vi "Prompt User for Init Type.vi"(8 "error in (no error)":errorcluster) -> (0 "error out":errorcluster, 3 "Path out":path)   [LabVIEW 2019, in "FPGA Addon System Explorer.lvlib"]
uses:
  FPGA Addon System Explorer.lvlib
panel:
  in  "New Instance?":bool
  in  "OK":bool
  in  "Path":path
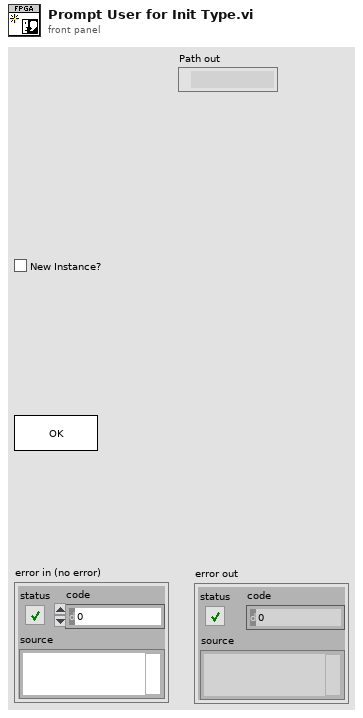
[diagram p1: front panel]
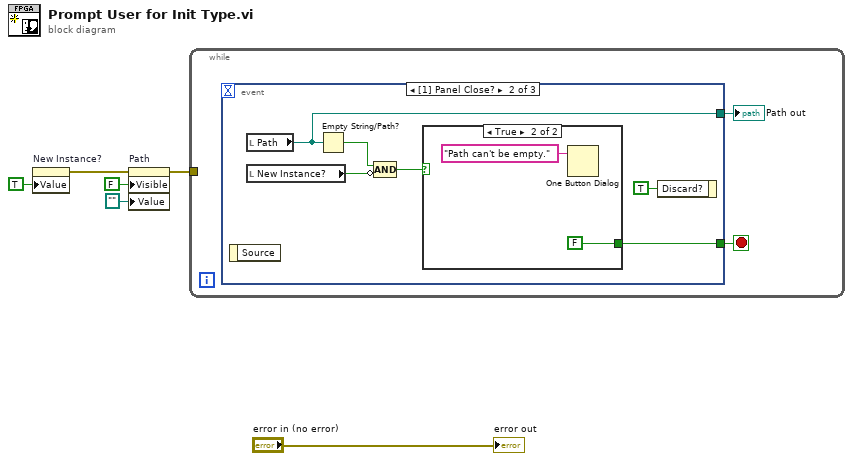
[diagram p0: block diagram]
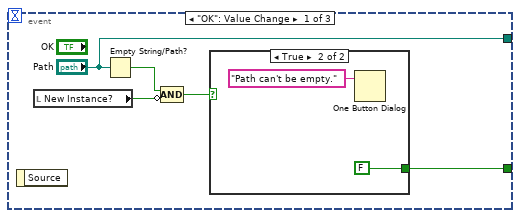
[diagram p2: hidden frame]
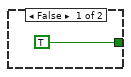
[diagram p3: hidden frame]
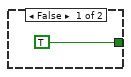
[diagram p4: hidden frame]
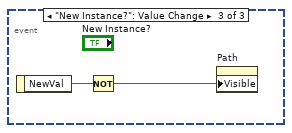
[diagram p5: hidden frame]
diagram:
  n1 = property on="New Instance?" class="Bool (strict)"("Value"=TRUE ("New Instance?")) -> (error out=w3:errorcluster)  [unwired: 2 in, 1 out]
  n2 = property on="Path" class="Path"(error in=w3, "Visible"=FALSE, "Value"=path "") -> (error out=w5:errorcluster)  [unwired: 1 in, 1 out]
  n3 = while {
    tunnel: w5 -> [_]
    stop <- w8 stop-if-true
    n4 = event shown="[1] Panel Close?" {
      selector: _ -> [_ _ _]
      dyn-events: _ -> [_ _ _]
      timeout: _ -> [_ _ _]
      tunnel: [w13 w22 _] -> w8
      tunnel: ["Path" w17 _] -> w7
      event "OK": Value Change {
        n5 = event-data() -> ()  [unwired: 1 in, 1 out]
        n6 = local read "New Instance?"() -> (w11:bool)
        n7 = Empty String/Path?(string/path="Path") -> (empty?=w10:bool)
        n8 = Compound Arithmetic op=AND(w10, invert w11) -> (w9:bool)
        n9 = case shown="True" w9 {
          tunnel: [TRUE FALSE] -> w13
          frame False {
          }
          frame True {
            n10 = One Button Dialog(message="Path can't be empty.") -> ()  [unwired: 1 in, 1 out]
          }
        }
      }
      event Panel Close? {
        n11 = event-data() -> ()  [unwired: 1 in, 1 out]
        n12 = local read "Path"() -> (w17:path)
        n13 = local read "New Instance?"() -> (w21:bool)
        n14 = Empty String/Path?(string/path=w17) -> (empty?=w20:bool)
        n15 = Compound Arithmetic op=AND(w20, invert w21) -> (w19:bool)
        n16 = case shown="True" w19 {
          tunnel: [TRUE FALSE] -> w22
          frame False {
          }
          frame True {
            n17 = One Button Dialog(message="Path can't be empty.") -> ()  [unwired: 1 in, 1 out]
          }
        }
        n18 = event-data("Discard?"=TRUE) -> ()  [unwired: 1 in, 1 out]
      }
      event "New Instance?": Value Change {
        n19 = event-data() -> ("NewVal"=w27:bool)  [unwired: 1 in]
        n20 = Not(x=w27) -> (.not. x?=w26:bool)
        n21 = property on="Path" class="Path"("Visible"=w26) -> ()  [unwired: 2 in, 2 out]
      }
    }
    "Path out" <- w7
  }
  "error out" <- "error in (no error)"
